vi "Equi-Ripple LowPass.vi"   [LabVIEW 2014, in "NI_AALBase.lvlib"]
doc: "Generates a lowpass FIR filter with equi-ripple characteristics using the Parks-McClellan algorithm and the <B># of taps</B>, <B>pass freq</B>, <B>stop freq</B>, and <B>sampling freq: fs</B>. The Equi-Ripple LowPass VI then applies a linear-phase, lowpass filter to the input sequence <B>X</B> using the Convolution VI to obtain <B>Filtered X</B>. Wire data to the <B>X</B> input to determine the polymorphic instance to use or manually select the instance."
uses:
  NI_AALBase.lvlib
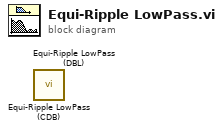
[diagram p0: block diagram]
diagram:
  n1 = call "Equi-Ripple LowPass (CDB).vi"() -> ()  [unwired: 6 in, 2 out]
  n2 = call "Equi-Ripple LowPass (DBL).vi"() -> ()  [unwired: 6 in, 2 out]
